vi "open select sample sheet.vi"(7 "Number of Sample Sheets":i32, 8 "error in (no error)":errorcluster, 9 "Worksheet Names":string[](array[string]), 10 "Active Sample Sheet":i32, 11 "NI_report in":refnum<class "NI_report.lvclass">) -> (0 "error out":errorcluster, 1 "Current Sample Sheet":string, 3 "NI_report out":refnum<class "NI_report.lvclass">, 4 "Select Worksheet Index":i32)   [LabVIEW 2016]
uses:
  <vilib>/Utility/NIReport.llb/NI_report.lvclass
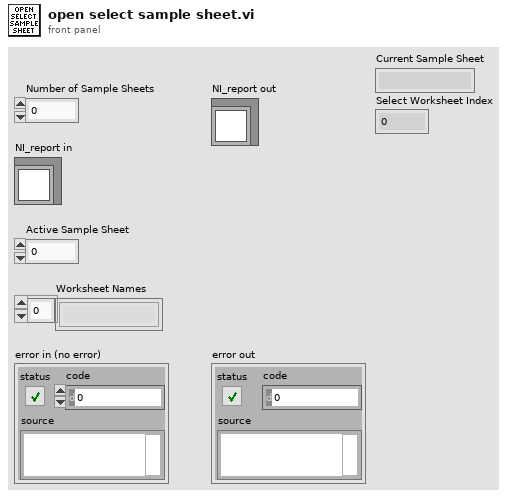
[diagram p1: front panel]
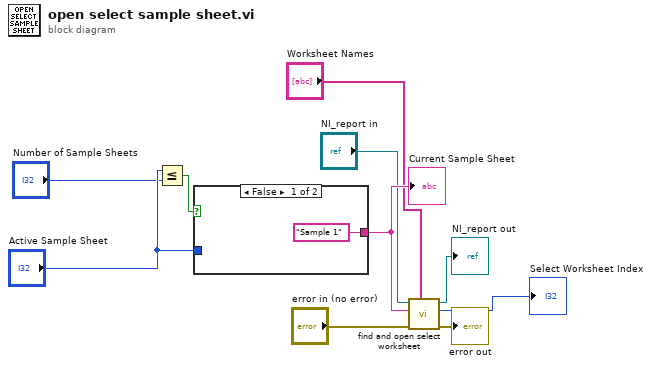
[diagram p0: block diagram]
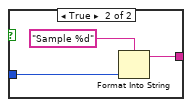
[diagram p2: hidden frame]
diagram:
  n1 = Less Or Equal?(x="Active Sample Sheet", y="Number of Sample Sheets") -> (x <= y?=w8:bool)
  n2 = case shown="False" w8 {
    tunnel: ["Sample 1" w14] -> w7
    tunnel: "Active Sample Sheet" -> [_ w13]
    frame False {
    }
    frame True {
      n3 = Format Into String(format string="Sample %d" ("Worksheet Name 1"), w13) -> (resulting string=w14:string)  [unwired: 2 in, 1 out]
    }
  }
  "Current Sample Sheet" <- w7
  n4 = call "find and open select worksheet.vi"("Worksheet Names"="Worksheet Names", "error in (no error)"="error in (no error)", "Worksheet Name in"=w7, "NI_report in"="NI_report in") -> ("error out"=→"error out":errorcluster, "Select Worksheet Index"=→"Select Worksheet Index":i32, "NI_report out"=→"NI_report out":refnum<class "NI_report.lvclass">)  [unwired: 5 in]
